vi "Ctor Device.vi"(8 "error in (no error)":errorcluster, 11 "Signal Generator in":refnum<class "Signal Generator.lvclass">) -> (0 "error out":errorcluster, 3 "Signal Generator out":refnum<class "Signal Generator.lvclass">)   [LabVIEW 2020, in "Signal Generator.lvlib" / "Signal Generator.lvclass"]
uses:
  Signal Generator.lvclass
  Ref Data.ctl
  Waveform Definition.ctl
  Waveform Type.ctl
  Signal Generator.lvclass/Signal Generator.ctl
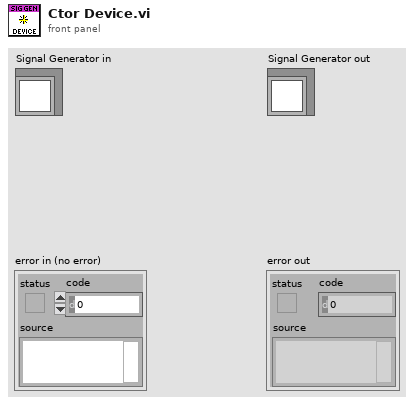
[diagram p1: front panel]
types:
  T1 = typedef "Signal Generator.lvlib/Signal Generator.lvclass/Ref Data.ctl" = cluster{"Waveform Definition":T2}
  T2 = typedef "Signal Generator.lvlib/Signal Generator.lvclass/Waveform Definition.ctl" = cluster{"Waveform Type":T3, "Frequency":dbl, "Amplitude":dbl}
  T3 = typedef "Signal Generator.lvlib/Signal Generator.lvclass/Waveform Type.ctl" = enum16{"Sine Wave", "Triangle Wave", "Square Wave", "Sawtooth Wave"}
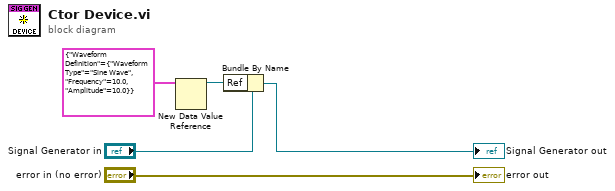
[diagram p0: block diagram]
diagram:
  n1 = New Data Value Reference(data value=T1 {"Waveform Definition"={"Waveform Type"=enum."Sine Wave", "Frequency"=10.0, "Amplitude"=10.0}} ("Ref Data")) -> (data value reference=w1:refnum<data-value>)  [unwired: 1 in, 1 out]
  n2 = Bundle By Name(cluster="Signal Generator in", "Ref"=w1) -> (→"Signal Generator out":refnum<class "Signal Generator.lvclass">)
  "error out" <- "error in (no error)"
